vi "set_stage (SubVI).vi"(0 "Tot Stage Arr":dbl[](array[numeric]), 1 "Volt vs pos array":cluster{dbl, dbl}[](array[cluster]), 2 "small amp":dbl=1.0 format="%0.2p", 3 "small amp freq":dbl=10.0 format="%0.2p", 4 "Add small amp?":bool, 5 "electrode arr":dbl[][](array[numeric]), 9 "electrodes task":refnum<k21>, 11 "electrodes task error":errorcluster, 12 "Num samples":i32, 13 "Use arb force?":bool, 14 "Electrode to sweep":i32) -> (10 "electrodes task 2":refnum<k21>, 15 "electrodes task error 2":errorcluster)   [LabVIEW 2014]
uses:
  <vilib>/DAQmx/write.llb/DAQmx Write (Analog 2D DBL NChan NSamp).vi
  <vilib>/measure/NI_MABase.lvlib
  <resource>/objmgr/daqmx.rc
panel:
  out "Waveform Graph":dbl[][](graph)
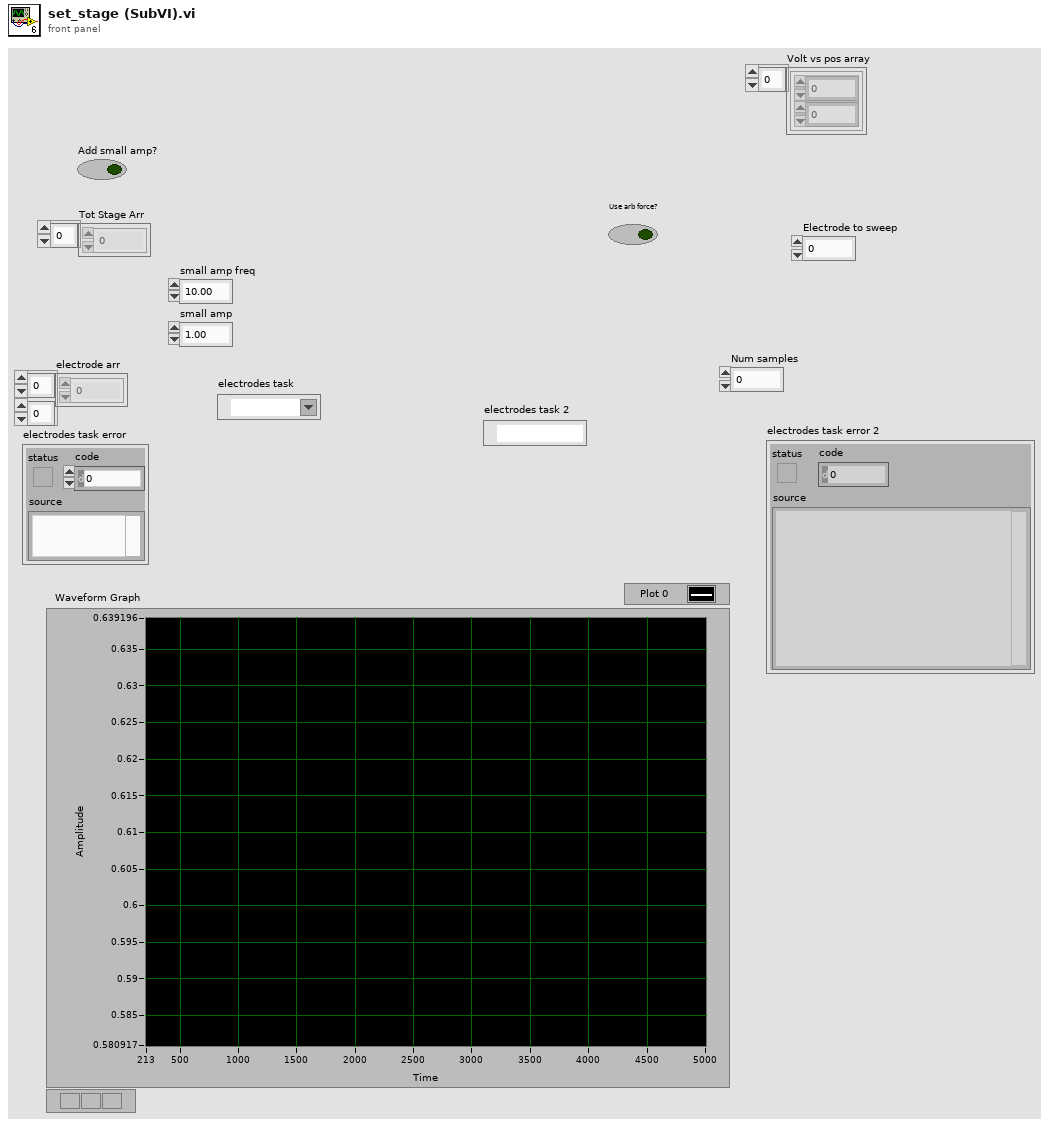
[diagram p1: front panel]
types:
  T1 = enum16{"Sine Wave", "Triangle Wave", "Square Wave", "Sawtooth Wave"}
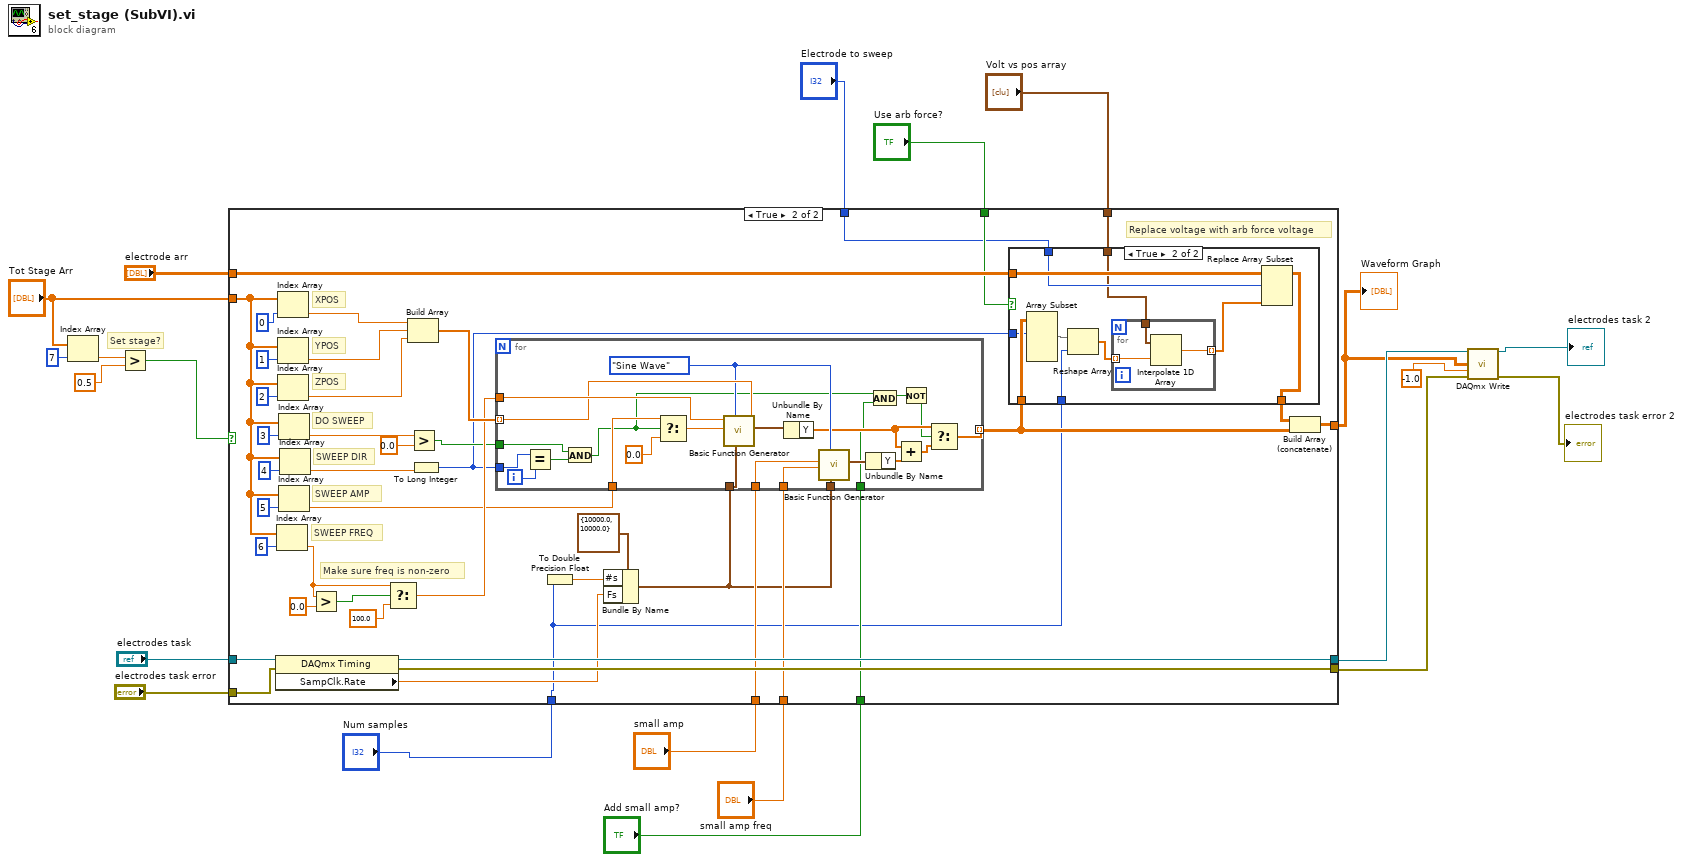
[diagram p0: block diagram]
diagram:
  # "Set stage?"
  n1 = Index Array(array="Tot Stage Arr", index=7) -> (element=w20:dbl)
  n2 = Greater?(x=w20, y=0.5) -> (0:w18:bool)
  n3 = case shown="True" w18 {
    tunnel: "electrode arr" -> [w24 w32]
    tunnel: [w24 w38] -> w8
    tunnel: "Tot Stage Arr" -> [_ w59]
    tunnel: "electrodes task" -> [w23 w54]
    tunnel: "electrodes task error" -> [w22 w53]
    tunnel: [w23 w52] -> w10
    tunnel: [w22 w51] -> w9
    tunnel: "Num samples" -> [_ w25]
    tunnel: "small amp freq" -> [_ w36]
    tunnel: "small amp" -> [_ w35]
    tunnel: "Add small amp?" -> [_ w33]
    tunnel: "Use arb force?" -> [_ w30]
    tunnel: "Electrode to sweep" -> [_ w29]
    tunnel: "Volt vs pos array" -> [_ w26]
    frame False {
    }
    frame True {
      # "Replace voltage with arb force voltage"
      # "Make sure freq is non-zero"
      # "SWEEP FREQ"
      # "SWEEP AMP"
      # "SWEEP DIR"
      # "DO SWEEP"
      # "ZPOS"
      # "YPOS"
      # "XPOS"
      n4 = property class="DAQmx Timing"(reference=w54, error in=w53) -> (reference out=w52:refnum<k21>, error out=w51:errorcluster, "SampClk.Rate"=w39:dbl)
      n5 = Index Array(array=w59, index=6) -> (element=w56:dbl)
      n6 = Index Array(array=w59, index=0) -> (element=w49:dbl)
      n7 = Index Array(array=w59, index=1) -> (element=w48:dbl)
      n8 = Index Array(array=w59, index=2) -> (element=w47:dbl)
      n9 = Index Array(array=w59, index=3) -> (element=w44:dbl)
      n10 = Index Array(array=w59, index=5) -> (element=w41:dbl)
      n11 = Index Array(array=w59, index=4) -> (element=w40:dbl)
      n12 = Greater?(x=w56, y=0.0) -> (0:w55:bool)
      n13 = Select(t=w56, s=w55, f=100.0) -> (s? t:f=w45:dbl)
      n14 = Build Array(w49, w48, w47) -> (w46:dbl[])
      n15 = Greater?(x=w44, y=0.0) -> (0:w42:bool)
      n16 = To Long Integer(number=w40) -> (32bit integer=w27:i32)
      n17 = To Double Precision Float(number=w25) -> (double precision float=w37:dbl)
      n18 = Bundle By Name(cluster=cluster{"Fs":dbl, "#s":dbl} {"Fs"=10000.0, "#s"=10000.0} ("sampling info"), "#s"=w37, "Fs"=w39) -> (w34:cluster{"Fs":dbl, "#s":dbl})
      n19 = for {
        tunnel: w46 -> [w103] mode=indexing
        tunnel: w45 -> [w104]
        tunnel: w27 -> [w99]
        tunnel: w34 -> [w98]
        tunnel: [w87] -> w28 mode=indexing
        tunnel: w42 -> [w95]
        tunnel: w41 -> [w94]
        tunnel: w36 -> [w91]
        tunnel: w35 -> [w90]
        tunnel: w34 -> [w88]
        tunnel: w33 -> [w83]
        i -> [w100]
        w89 = T1."Sine Wave" ("signal type")
        n20 = Equal?(x=w99, y=w100) -> (x = y?=w96:bool)
        n21 = And(x=w95, y=w96) -> (x .and. y?=w84:bool)
        n22 = Select(t=w94, s=w84, f=0.0) -> (s? t:f=w102:dbl)
        n23 = call <vilib>:"Basic Function Generator.vi"("offset"=w103, "sampling info"=w98, "signal type"=w89, "amplitude"=w102, "frequency"=w104) -> ("signal out"=w97:waveform(dbl))  [unwired: 4 in, 2 out]
        n24 = Unbundle By Name(w97) -> ("Y"=w85:dbl[])
        n25 = call <vilib>:"Basic Function Generator.vi"("sampling info"=w88, "signal type"=w89, "amplitude"=w90, "frequency"=w91) -> ("signal out"=w93:waveform(dbl))  [unwired: 5 in, 2 out]
        n26 = Unbundle By Name(w93) -> ("Y"=w92:dbl[])
        n27 = And(x=w84, y=w83) -> (x .and. y?=w81:bool)
        n28 = Add(x=w85, y=w92) -> (x+y=w86:dbl[])
        n29 = Not(x=w81) -> (.not. x?=w82:bool)
        n30 = Select(t=w85, s=w82, f=w86) -> (s? t:f=w87:dbl[])
      }
      n31 = case shown="True" w30 {
        tunnel: w32 -> [w67 w77]
        tunnel: [w67 w76] -> w31
        tunnel: w29 -> [_ w75]
        tunnel: w28 -> [_ w74]
        tunnel: w27 -> [_ w73]
        tunnel: w26 -> [_ w69]
        tunnel: w25 -> [_ w68]
        frame False {
        }
        frame True {
          n32 = Array Subset(array=w74, index (row)=w73) -> (w72:dbl[][])  [unwired: 3 in]
          n33 = Reshape Array(w72, w68) -> (w71:dbl[])
          n34 = for {
            tunnel: w71 -> [w80] mode=indexing
            tunnel: [w79] -> w70 mode=indexing
            tunnel: w69 -> [w78]
            n35 = Interpolate 1D Array(1:w80, 2:w78) -> (0:w79:dbl)
          }
          n36 = Replace Array Subset(array=w77, new element=w70, index (row)=w75) -> (w76:dbl[][])  [unwired: 1 in]
        }
      }
      n37 = Build Array (concatenate)(w31, w28) -> (w38:dbl[][])
    }
  }
  "Waveform Graph" <- w8
  n38 = call-poly <vilib>:"DAQmx Write.vi"("task/channels in"=w10, "data"=w8, "timeout"=-1.0, "error in"=w9) -> ("task out"=→"electrodes task 2":refnum<k21>, "error out"=→"electrodes task error 2":errorcluster)  [unwired: 9 in, 1 out]
